vi "flush file buffers.vi"(8 "error in":errorcluster, 10 "Flush interval (s)":dbl=60.0 format="%.2f", 11 "refnum":refnum<file>) -> (0 "error out":errorcluster, 3 "dup refnum":refnum<file>)   [LabVIEW 2015]
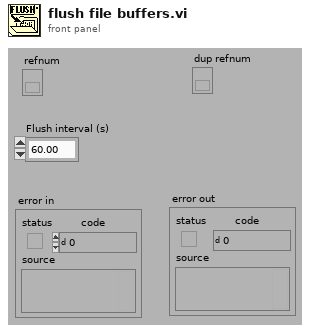
[diagram p1: front panel]
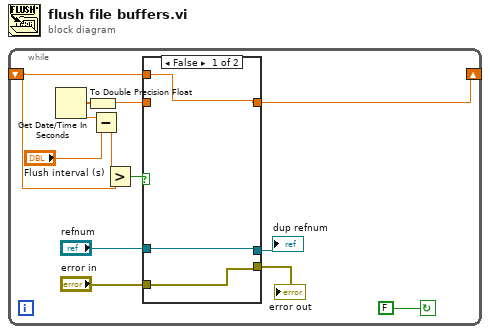
[diagram p0: block diagram]
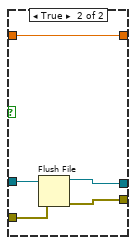
[diagram p2: hidden frame]
diagram:
  n1 = while {
    shift-right: [w8] -> _
    shift-left: _ -> [w2]
    stop <- FALSE continue-if-true
    n2 = Get Date/Time In Seconds() -> (seconds since 1Jan1904=w1:timestamp)
    n3 = To Double Precision Float(number=w1) -> (double precision float=w7:dbl)
    n4 = Subtract(x=w7, y="Flush interval (s)") -> (x-y=w10:dbl)
    n5 = Greater?(x=w10, y=w2) -> (0:w9:bool)
    n6 = case shown="False" w9 {
      tunnel: [w15 w20] -> w8
      tunnel: w7 -> [_ w20]
      tunnel: w2 -> [w15 _]
      tunnel: "refnum" -> [w14 w19]
      tunnel: [w14 w18] -> w5
      tunnel: "error in" -> [w13 w17]
      tunnel: [w13 w16] -> w3
      frame False {
      }
      frame True {
        n7 = Flush File(refnum=w19, error in=w17) -> (refnum out=w18:refnum<file>, error out=w16:errorcluster)
      }
    }
    "error out" <- w3
    "dup refnum" <- w5
  }
